vi "PH_DataViewer.set Img Op GUI elements.vi"(0 "i ref in":refnum<vi>, 2 "Img Operator Data":T2={"Instance"="N/A", "Snapshot: Date"="N/A", "Snapshot: Time"="N/A", "Calibration"={"Status"=0, "Calibration data - Version 1"={"Date"="", "Time"="", "Cam Settings"={"Serial Number"=0.0, "Gain"=0, "Brightness"=0, "Shutter"=0, "Cam Error"=FALSE, "Mode"=0}, "Background Image"={"Image"=[], "Image Error"=FALSE}, "Linear Calibration"={"Calibration Factor"=0.0, "not mm or mrad"=FALSE}, "Energy Calibration"={"Calibration Factor"=0.0, "no mJ"=FALSE}}}, "Position Analysis"={"on"=FALSE, "exp - X"=0, "exp - Y"=0, "focal length [mm]"=0.0, "Magnification"=0.0, "Delta"=0.0, "Theta"=0.0, "Tolerance"=0.0, "Type"=FALSE}, "Beam Analysis"={"on"=FALSE, "Data"={"CoG-x"=0.0, "CoG-y"=0.0, "Maj Dim"=0.0, "Min Dim"=0.0, "Ellipticity"=0.0, "Azimuth Angle [rad]"=0.0, "Azi Angle rel to Maj?"=FALSE}, "Method"=FALSE, "Steps"=3, "Factor"=3, "ROI"={"Left"=0, "Top"=0, "Right"=0, "Bottom"=0}}, "Cam Settings"={"Serial Number"=0.0, "Gain"=0, "Brightness"=0, "Shutter"=0, "Cam Info Failure"=FALSE, "Mode"=0}, "Energy"={"on"=FALSE, "expected value [mJ]"=0.0, "Tolerance [%]"=0.0, "State"=0, "Energy [mJ]"=0.0, "Unit"=""}, "Image"=[], "Final Image"={"BI Subtraction Failure"=FALSE}, "Trace Analysis"={"on"=FALSE, "Fit on"=FALSE, "Maj FWHM"=0.0, "Min FWHM"=0.0, "Maj Fit Order"=0, "Min Fit Order"=0, "No Offset"=FALSE, "Maj 99%"=0.0, "Min 99%"=0.0, "Traces"=[]}} {"Energy"."State" items=["no info", "off/false", "on/true", "Failure", "Alarm"]; "Cam Settings"."Serial Number" format="%#_12g"; "Calibration"."Calibration data - Version 1"."Cam Settings"."Serial Number" format="%#_12g"; "Calibration"."Status" items=["no info", "off/false", "on/true", "Failure", "Alarm"]}, 5 "error in (no error)":errorcluster) -> (14 "i ref out":refnum<vi>, 19 "error out":errorcluster)   [LabVIEW 2014, in "PH_DataViewer.lvlib"]
doc: "This VI indicates the results of the Image Operator"
uses:
  PH_DataViewer.lvlib
  PH_ImageOperator.Data.ctl
  PH_DataViewer.Device State.ctl
  PH_ImageCalibrator/PH_ImageCalibrator.Calibration Data - Version 1.ctl
  PH_ImageOperator/PH_ImageOperator.Beam Analysis Data.ctl
  <vilib>/vision/Image Controls.llb/IMAQ Image.ctl
  <vilib>/vision/NI_Vision_Development_Module.lvlib
  PH_ImageOperator/PH_ImageOperator.lvlib
  PH_ImageCalibrator/PH_ImageCalibrator.lvlib
panel:
  in  "Cam Settings Template":T1 caption="Settings" {"Serial Number" format="%#_15g"}
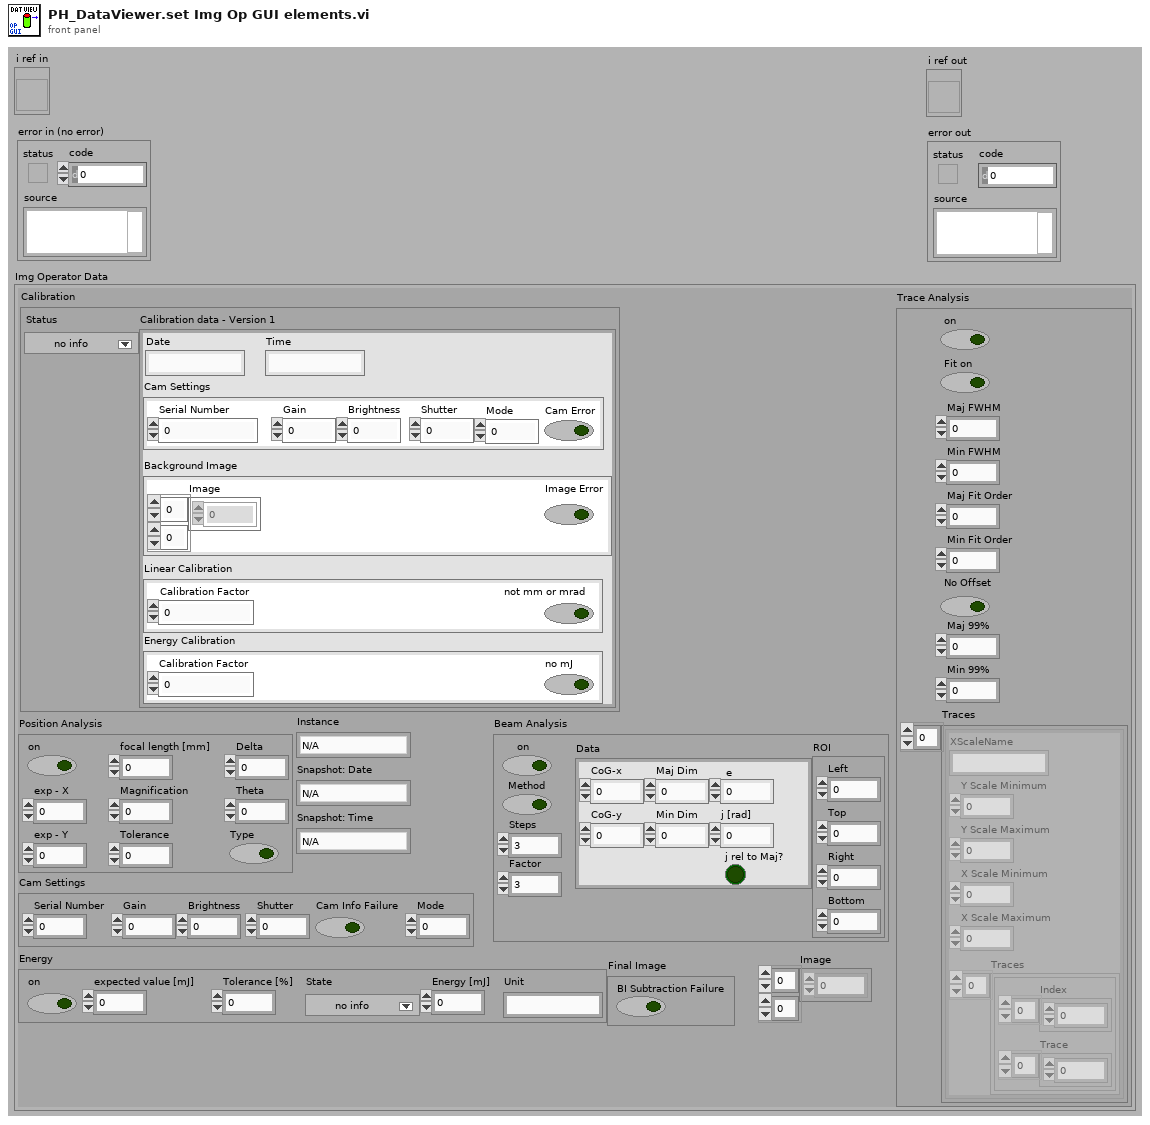
[diagram p1: front panel]
types:
  T1 = cluster{"Serial Number":dbl, "Gain":i32, "Brightness":i32, "Shutter":i32, "Mode":i32}
  T2 = typedef "PH_DataViewer.lvlib/PH_ImageOperator.Data.ctl" = cluster{"Instance":string, "Snapshot: Date":string, "Snapshot: Time":string, "Calibration":cluster{"Status":T3, "Calibration data - Version 1":T4}, "Position Analysis":cluster{"on":bool, "exp - X":i32, "exp - Y":i32, "focal length [mm]":dbl, "Magnification":dbl, "Delta":dbl, "Theta":dbl, "Tolerance":dbl, "Type":bool}, "Beam Analysis":cluster{"on":bool, "Data":T5, "Method":bool, "Steps":i32, "Factor":i32, "ROI":cluster{"Left":i32, "Top":i32, "Right":i32, "Bottom":i32}}, "Cam Settings":cluster{"Serial Number":dbl, "Gain":i32, "Brightness":i32, "Shutter":i32, "Cam Info Failure":bool, "Mode":i32}, "Energy":cluster{"on":bool, "expected value [mJ]":dbl, "Tolerance [%]":dbl, "State":T3, "Energy [mJ]":dbl, "Unit":string}, "Image":dbl[][], "Final Image":cluster{"BI Subtraction Failure":bool}, "Trace Analysis":cluster{"on":bool, "Fit on":bool, "Maj FWHM":dbl, "Min FWHM":dbl, "Maj Fit Order":i32, "Min Fit Order":i32, "No Offset":bool, "Maj 99%":dbl, "Min 99%":dbl, "Traces":cluster{"XScaleName":string, "Y Scale Minimum":sgl, "Y Scale Maximum":sgl, "X Scale Minimum":sgl, "X Scale Maximum":sgl, "Traces":cluster{"Index":sgl[], "Trace":dbl[]}[]}[]}}
  T3 = typedef "PH_DataViewer.lvlib/PH_DataViewer.Device State.ctl" = i32
  T4 = typedef "PH_ImageCalibrator.lvlib/PH_ImageCalibrator.Calibration Data - Version 1.ctl" = cluster{"Date":string, "Time":string, "Cam Settings":cluster{"Serial Number":dbl, "Gain":i32, "Brightness":i32, "Shutter":i32, "Cam Error":bool, "Mode":i32}, "Background Image":cluster{"Image":dbl[][], "Image Error":bool}, "Linear Calibration":cluster{"Calibration Factor":dbl, "not mm or mrad":bool}, "Energy Calibration":cluster{"Calibration Factor":dbl, "no mJ":bool}}
  T5 = typedef "PH_ImageOperator.lvlib/PH_ImageOperator.Beam Analysis Data.ctl" = cluster{"CoG-x":sgl, "CoG-y":sgl, "Maj Dim":dbl, "Min Dim":dbl, "Ellipticity":dbl, "Azimuth Angle [rad]":dbl, "Azi Angle rel to Maj?":bool}
  T6 = typedef "PH_DataViewer.lvlib/PH_DataViewer.i attribute.ctl" = cluster{"Images":cluster{"CAM":cluster{string, u32}, "BACKGROUND":cluster{string, u32}, "OPERATOR":cluster{string, u32}}, "Cam Operator GUI Refs":cluster{"Date Operators":refnum<vi>, "Time Operators":refnum<vi>, "Status Cali Data":refnum<vi>, "Calibration data":refnum<vi>, "Background Image":refnum<vi>, "Bg subtracted":refnum<vi>, "Op Image":refnum<vi>, "Cam Settings Operator":refnum<vi>, "Energy on":refnum<vi>, "exp Energy":refnum<vi>, "Energy":refnum<vi>, "Beam Analysis":refnum<vi>, "Analysis Type":refnum<vi>, "BA: Steps":refnum<vi>, "BA: Factor for ROI":refnum<vi>, "CoG - X":refnum<vi>, "CoG - Y":refnum<vi>, "Maj Diam":refnum<vi>, "Min Diam":refnum<vi>, "Phi":refnum<vi>, "Epsilon":refnum<vi>, "Phi rel to maj":refnum<vi>, "Position":refnum<vi>, "Position Type":refnum<vi>, "exp - X":refnum<vi>, "exp - Y":refnum<vi>, "Magni":refnum<vi>, "Foc Length":refnum<vi>, "Delta":refnum<vi>, "Theta":refnum<vi>, "Fit Gauss":refnum<vi>, "Maj Fit Order":refnum<vi>, "Min Fit Order":refnum<vi>, "Maj FWHM":refnum<vi>, "Min FWHM":refnum<vi>, "Maj 1 %":refnum<vi>, "Min 1 %":refnum<vi>}}
  T7 = cluster{"Date Operators":refnum<vi>, "Time Operators":refnum<vi>, "Status Cali Data":refnum<vi>, "Calibration data":refnum<vi>, "Background Image":refnum<vi>, "Bg subtracted":refnum<vi>, "Op Image":refnum<vi>, "Cam Settings Operator":refnum<vi>, "Energy on":refnum<vi>, "exp Energy":refnum<vi>, "Energy":refnum<vi>, "Beam Analysis":refnum<vi>, "Analysis Type":refnum<vi>, "BA: Steps":refnum<vi>, "BA: Factor for ROI":refnum<vi>, "CoG - X":refnum<vi>, "CoG - Y":refnum<vi>, "Maj Diam":refnum<vi>, "Min Diam":refnum<vi>, "Phi":refnum<vi>, "Epsilon":refnum<vi>, "Phi rel to maj":refnum<vi>, "Position":refnum<vi>, "Position Type":refnum<vi>, "exp - X":refnum<vi>, "exp - Y":refnum<vi>, "Magni":refnum<vi>, "Foc Length":refnum<vi>, "Delta":refnum<vi>, "Theta":refnum<vi>, "Fit Gauss":refnum<vi>, "Maj Fit Order":refnum<vi>, "Min Fit Order":refnum<vi>, "Maj FWHM":refnum<vi>, "Min FWHM":refnum<vi>, "Maj 1 %":refnum<vi>, "Min 1 %":refnum<vi>}
  T8 = typedef "IMAQ Image.ctl" = refnum<image>
  T9 = cluster{"Date Operators":bool, "Time Operators":bool, "Status Cali Data":bool, "Calibration data":bool, "Background Image":bool, "Bg subtracted":bool, "Op Image":bool, "Cam Settings Operator":bool, "Energy on":bool, "exp Energy":bool, "Energy":bool, "Beam Analysis":bool, "Analysis Type":bool, "BA: Steps":bool, "BA: Factor for ROI":bool, "CoG - X":bool, "CoG - Y":bool, "Maj Diam":bool, "Min Diam":bool, "Phi":bool, "Epsilon":bool, "Phi rel to maj":bool, "Position":bool, "Position Type":bool, "exp - X":bool, "exp - Y":bool, "Magni":bool, "Foc Length":bool, "Delta":bool, "Theta":bool, "Fit Gauss":bool, "Maj Fit Order":bool, "Min Fit Order":bool, "Maj FWHM":bool, "Min FWHM":bool, "Maj 1 %":bool, "Min 1 %":bool}
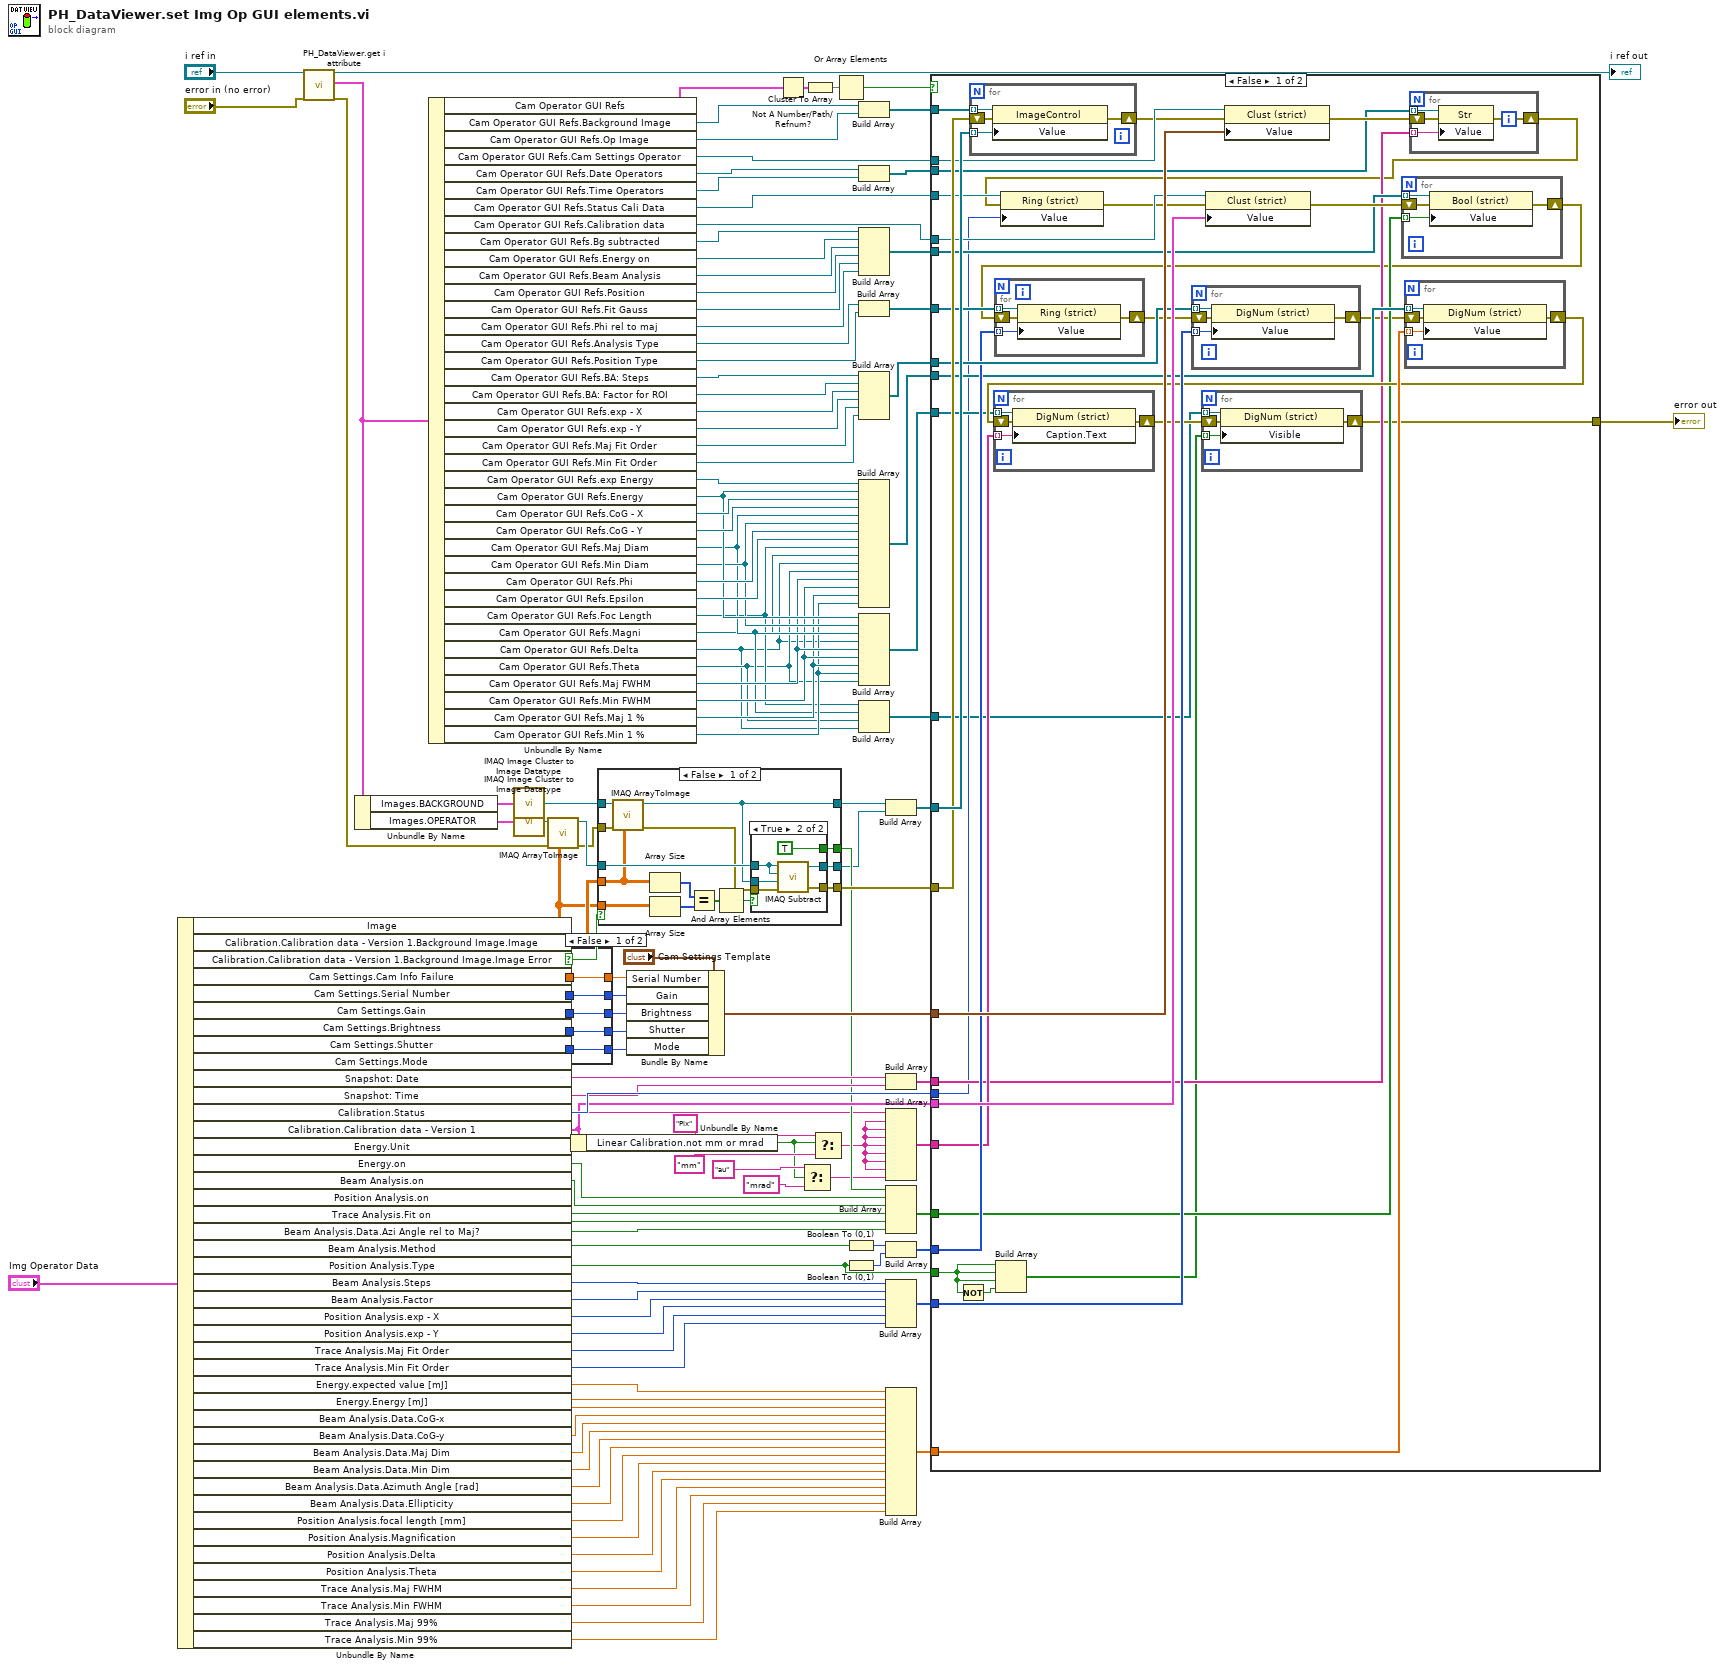
[diagram p0: block diagram]
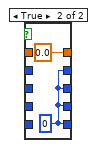
[diagram p3: hidden frame]
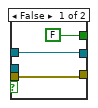
[diagram p4: hidden frame]
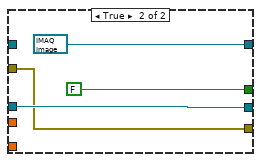
[diagram p5: hidden frame]
diagram:
  n1 = Unbundle By Name("Img Operator Data") -> ("Image"=w100:dbl[][], "Calibration.Calibration data - Version 1.Background Image.Image"=w101:dbl[][], "Calibration.Calibration data - Version 1.Background Image.Image Error"=w111:bool, "Cam Settings.Cam Info Failure"=w119:bool, "Cam Settings.Serial Number"=w120:dbl, "Cam Settings.Gain"=w122:i32, "Cam Settings.Brightness"=w124:i32, "Cam Settings.Shutter"=w126:i32, "Cam Settings.Mode"=w128:i32, "Snapshot: Date"=w64:string, "Snapshot: Time"=w65:string, "Calibration.Status"=w102:T3, "Calibration.Calibration data - Version 1"=w83:T4, "Energy.Unit"=w11:string, "Energy.on"=w77:bool, "Beam Analysis.on"=w78:bool, "Position Analysis.on"=w79:bool, "Trace Analysis.Fit on"=w80:bool, "Beam Analysis.Data.Azi Angle rel to Maj?"=w70:bool, "Beam Analysis.Method"=w96:bool, "Position Analysis.Type"=w1:bool, "Beam Analysis.Steps"=w49:i32, "Beam Analysis.Factor"=w50:i32, "Position Analysis.exp - X"=w32:i32, "Position Analysis.exp - Y"=w31:i32, "Trace Analysis.Maj Fit Order"=w30:i32, "Trace Analysis.Min Fit Order"=w29:i32, "Energy.expected value [mJ]"=w45:dbl, "Energy.Energy [mJ]"=w46:dbl, "Beam Analysis.Data.CoG-x"=w91:sgl, "Beam Analysis.Data.CoG-y"=w39:sgl, "Beam Analysis.Data.Maj Dim"=w90:dbl, "Beam Analysis.Data.Min Dim"=w89:dbl, "Beam Analysis.Data.Azimuth Angle [rad]"=w88:dbl, "Beam Analysis.Data.Ellipticity"=w87:dbl, "Position Analysis.focal length [mm]"=w24:dbl, "Position Analysis.Magnification"=w23:dbl, "Position Analysis.Delta"=w22:dbl, "Position Analysis.Theta"=w21:dbl, "Trace Analysis.Maj FWHM"=w20:dbl, "Trace Analysis.Min FWHM"=w19:dbl, "Trace Analysis.Maj 99%"=w18:dbl, "Trace Analysis.Min 99%"=w17:dbl)
  n2 = call "PH_DataViewer.get i attribute.vi"("i ref in"="i ref in", "error in (no error)"="error in (no error)") -> ("i ref out"=→"i ref out":refnum<vi>, "i attribute"=w99:T6, "error out"=w113:errorcluster)  [unwired: 15 in]
  n3 = Unbundle By Name(w99) -> ("Images.BACKGROUND"=w98:cluster{string, u32}, "Images.OPERATOR"=w97:cluster{string, u32})
  n4 = Unbundle By Name(w99) -> ("Cam Operator GUI Refs"=w110:T7, "Cam Operator GUI Refs.Background Image"=w60:refnum<vi>, "Cam Operator GUI Refs.Op Image"=w59:refnum<vi>, "Cam Operator GUI Refs.Cam Settings Operator"=w106:refnum<vi>, "Cam Operator GUI Refs.Date Operators"=w68:refnum<vi>, "Cam Operator GUI Refs.Time Operators"=w67:refnum<vi>, "Cam Operator GUI Refs.Status Cali Data"=w40:refnum<vi>, "Cam Operator GUI Refs.Calibration data"=w105:refnum<vi>, "Cam Operator GUI Refs.Bg subtracted"=w62:refnum<vi>, "Cam Operator GUI Refs.Energy on"=w75:refnum<vi>, "Cam Operator GUI Refs.Beam Analysis"=w74:refnum<vi>, "Cam Operator GUI Refs.Position"=w73:refnum<vi>, "Cam Operator GUI Refs.Fit Gauss"=w72:refnum<vi>, "Cam Operator GUI Refs.Phi rel to maj"=w69:refnum<vi>, "Cam Operator GUI Refs.Analysis Type"=w34:refnum<vi>, "Cam Operator GUI Refs.Position Type"=w35:refnum<vi>, "Cam Operator GUI Refs.BA: Steps"=w53:refnum<vi>, "Cam Operator GUI Refs.BA: Factor for ROI"=w52:refnum<vi>, "Cam Operator GUI Refs.exp - X"=w28:refnum<vi>, "Cam Operator GUI Refs.exp - Y"=w27:refnum<vi>, "Cam Operator GUI Refs.Maj Fit Order"=w26:refnum<vi>, "Cam Operator GUI Refs.Min Fit Order"=w25:refnum<vi>, "Cam Operator GUI Refs.exp Energy"=w47:refnum<vi>, "Cam Operator GUI Refs.Energy"=w43:refnum<vi>, "Cam Operator GUI Refs.CoG - X"=w94:refnum<vi>, "Cam Operator GUI Refs.CoG - Y"=w54:refnum<vi>, "Cam Operator GUI Refs.Maj Diam"=w41:refnum<vi>, "Cam Operator GUI Refs.Min Diam"=w42:refnum<vi>, "Cam Operator GUI Refs.Phi"=w93:refnum<vi>, "Cam Operator GUI Refs.Epsilon"=w92:refnum<vi>, "Cam Operator GUI Refs.Foc Length"=w6:refnum<vi>, "Cam Operator GUI Refs.Magni"=w5:refnum<vi>, "Cam Operator GUI Refs.Delta"=w3:refnum<vi>, "Cam Operator GUI Refs.Theta"=w4:refnum<vi>, "Cam Operator GUI Refs.Maj FWHM"=w16:refnum<vi>, "Cam Operator GUI Refs.Min FWHM"=w15:refnum<vi>, "Cam Operator GUI Refs.Maj 1 %"=w14:refnum<vi>, "Cam Operator GUI Refs.Min 1 %"=w13:refnum<vi>)
  n5 = call <vilib>:"IMAQ Image Cluster to Image Datatype.vi"("Image"=w98) -> ("Image (dup)"=w116:T8)
  n6 = call <vilib>:"IMAQ Image Cluster to Image Datatype.vi"("Image"=w97) -> ("Image (dup)"=w118:T8)
  n7 = call "IMAQ ArrayToImage"("Image Pixels (Float)"=w100, "error in (no error)"=w113, "Image"=w118) -> ("error out"=w114:errorcluster, "Image Out"=w117:T8)  [unwired: 7 in]
  n8 = case shown="False" w119 {
    tunnel: w120 -> [w137 _]
    tunnel: [w137 0.0 ("Serial Number")] -> w121
    tunnel: [w136 w138] -> w123
    tunnel: w122 -> [w136 _]
    tunnel: [w135 w138] -> w125
    tunnel: w124 -> [w135 _]
    tunnel: [w134 w138] -> w127
    tunnel: w126 -> [w134 _]
    tunnel: [w133 w138] -> w129
    tunnel: w128 -> [w133 _]
    frame False {
    }
    frame True {
      w138 = 0 ("Gain")
    }
  }
  n9 = Unbundle By Name(w83) -> ("Linear Calibration.not mm or mrad"=w8:bool)
  n10 = case shown="False" w111 {
    tunnel: w101 -> [w145 _]
    tunnel: [w151 T8 refnum ("Image Out")] -> w55
    tunnel: w116 -> [w153 _]
    tunnel: w117 -> [w152 w165]
    tunnel: [w150 w165] -> w57
    tunnel: [w149 FALSE] -> w61
    tunnel: w114 -> [w148 w163]
    tunnel: [w146 w163] -> w104
    tunnel: w100 -> [w144 _]
    frame False {
      n11 = call "IMAQ ArrayToImage"("Image Pixels (Float)"=w145, "error in (no error)"=w148, "Image"=w153) -> ("error out"=w147:errorcluster, "Image Out"=w151:T8)  [unwired: 7 in]
      n12 = Array Size(array=w145) -> (size(s)=w142:i32[])
      n13 = Array Size(array=w144) -> (size(s)=w143:i32[])
      n14 = Equal?(x=w142, y=w143) -> (x = y?=w141:bool[])
      n15 = And Array Elements(Boolean array=w141) -> (logical AND=w140:bool)
      n16 = case shown="True" w140 {
        tunnel: w152 -> [w155 w162]
        tunnel: w151 -> [_ w161]
        tunnel: [w155 w160] -> w150
        tunnel: [FALSE TRUE] -> w149
        tunnel: w147 -> [w154 w158]
        tunnel: [w154 w157] -> w146
        frame False {
        }
        frame True {
          n17 = call "IMAQ Subtract"("Image Src A"=w162, "Image Dst"=w162, "Image Src B"=w161, "error in (no error)"=w158) -> ("Image Dst Out"=w160:T8, "error out"=w157:errorcluster)  [unwired: 3 in]
        }
      }
    }
    frame True {
    }
  }
  n18 = Bundle By Name(cluster="Cam Settings Template", "Serial Number"=w121, "Gain"=w123, "Brightness"=w125, "Shutter"=w127, "Mode"=w129) -> (w103:T1)
  n19 = Not A Number/Path/Refnum?(number/path/refnum=w110) -> (NaN/Path/Refnum?=w108:T9)
  n20 = Select(t="au", s=w8, f="mrad") -> (s? t:f=w7:string)
  n21 = Cluster To Array(cluster=w108) -> (array=w109:bool[])
  n22 = Select(t="Pix", s=w8, f="mm") -> (s? t:f=w12:string)
  n23 = Or Array Elements(Boolean array=w109) -> (logical OR=w107:bool)
  n24 = Boolean To (0,1)(Boolean=w96) -> (0, 1=w37:i16)
  n25 = Boolean To (0,1)(Boolean=w1) -> (0, 1=w38:i16)
  n26 = Build Array(w60, w59) -> (w58:refnum<vi>[])
  n27 = Build Array(w68, w67) -> (w66:refnum<vi>[])
  n28 = Build Array(w62, w75, w74, w73, w72, w69) -> (w71:refnum<vi>[])
  n29 = Build Array(w34, w35) -> (w33:refnum<vi>[])
  n30 = Build Array(w53, w52, w28, w27, w26, w25) -> (w51:refnum<vi>[])
  n31 = Build Array(w47, w43, w94, w54, w41, w42, w93, w92, w6, w5, w3, w4, w16, w15, w14, w13) -> (w85:refnum<vi>[])
  n32 = Build Array(w43, w42, w41, w3, w16, w15, w14, w13, w4) -> (w84:refnum<vi>[])
  n33 = Build Array(w6, w5, w4, w3) -> (w2:refnum<vi>[])
  n34 = Build Array(w55, w57) -> (w56:T8[])
  n35 = Build Array(w64, w65) -> (w63:string[])
  n36 = Build Array(w11, w12, w12, w12, w12, w12, w12, w12, w7) -> (w44:string[])
  n37 = Build Array(w61, w77, w78, w79, w80, w70) -> (w76:bool[])
  n38 = Build Array(w37, w38) -> (w36:i16[])
  n39 = Build Array(w49, w50, w32, w31, w30, w29) -> (w48:i32[])
  n40 = Build Array(w45, w46, w91, w39, w90, w89, w88, w87, w24, w23, w22, w21, w20, w19, w18, w17) -> (w86:dbl[])
  n41 = case shown="False" w107 {
    tunnel: w58 -> [w177 _]
    tunnel: w106 -> [w200 _]
    tunnel: w40 -> [w197 _]
    tunnel: w105 -> [w196 _]
    tunnel: w56 -> [w202 _]
    tunnel: w104 -> [w201 w235]
    tunnel: w103 -> [w199 _]
    tunnel: w102 -> [w174 _]
    tunnel: w83 -> [w195 _]
    tunnel: w48 -> [w189 _]
    tunnel: w33 -> [w193 _]
    tunnel: w51 -> [w192 _]
    tunnel: w36 -> [w190 _]
    tunnel: [w171 w235] -> w95
    tunnel: w86 -> [w188 _]
    tunnel: w85 -> [w187 _]
    tunnel: w84 -> [w185 _]
    tunnel: w44 -> [w184 _]
    tunnel: w76 -> [w182 _]
    tunnel: w71 -> [w183 _]
    tunnel: w66 -> [w181 _]
    tunnel: w63 -> [w180 _]
    tunnel: w2 -> [w170 _]
    tunnel: w1 -> [w169 _]
    frame False {
      n42 = Not(x=w169) -> (.not. x?=w168:bool)
      n43 = for {
        tunnel: w202 -> [w218] mode=indexing
        shift-right: [w216] -> w179
        shift-left: w201 -> [w217]
        tunnel: w177 -> [w215] mode=indexing
        n44 = property class="ImageControl"(reference=w215, error in=w217, "Value"=w218) -> (error out=w216:errorcluster)  [unwired: 1 out]
      }
      n45 = Build Array(w169, w169, w169, w168) -> (w167:bool[])
      n46 = property class="Clust (strict)"(reference=w200, error in=w179, "Value"=w199) -> (error out=w198:errorcluster)  [unwired: 1 out]
      n47 = for {
        tunnel: w180 -> [w221] mode=indexing
        shift-right: [w220] -> w173
        shift-left: w198 -> [w222]
        tunnel: w181 -> [w219] mode=indexing
        n48 = property class="Str"(reference=w219, error in=w222, "Value"=w221) -> (error out=w220:errorcluster)  [unwired: 1 out]
      }
      n49 = property class="Ring (strict)"(reference=w197, error in=w173, "Value"=w174) -> (error out=w178:errorcluster)  [unwired: 1 out]
      n50 = property class="Clust (strict)"(reference=w196, error in=w178, "Value"=w195) -> (error out=w194:errorcluster)  [unwired: 1 out]
      n51 = for {
        shift-right: [w226] -> w175
        shift-left: w194 -> [w225]
        tunnel: w183 -> [w224] mode=indexing
        tunnel: w182 -> [w223] mode=indexing
        n52 = property class="Bool (strict)"(reference=w224, error in=w225, "Value"=w223) -> (error out=w226:errorcluster)  [unwired: 1 out]
      }
      n53 = for {
        tunnel: w193 -> [w210] mode=indexing
        tunnel: w190 -> [w208] mode=indexing
        shift-right: [w209] -> w191
        shift-left: w175 -> [w207]
        n54 = property class="Ring (strict)"(reference=w210, error in=w207, "Value"=w208) -> (error out=w209:errorcluster)  [unwired: 1 out]
      }
      n55 = for {
        tunnel: w192 -> [w214] mode=indexing
        tunnel: w189 -> [w212] mode=indexing
        shift-right: [w211] -> w176
        shift-left: w191 -> [w213]
        n56 = property class="DigNum (strict)"(reference=w214, error in=w213, "Value"=w212) -> (error out=w211:errorcluster)  [unwired: 1 out]
      }
      n57 = for {
        shift-right: [w233] -> w186
        shift-left: w176 -> [w234]
        tunnel: w187 -> [w232] mode=indexing
        tunnel: w188 -> [w231] mode=indexing
        n58 = property class="DigNum (strict)"(reference=w232, error in=w234, "Value"=w231) -> (error out=w233:errorcluster)  [unwired: 1 out]
      }
      n59 = for {
        shift-right: [w229] -> w172
        shift-left: w186 -> [w230]
        tunnel: w185 -> [w228] mode=indexing
        tunnel: w184 -> [w227] mode=indexing
        n60 = property class="DigNum (strict)"(reference=w228, error in=w230, "Caption.Text"=w227) -> (error out=w229:errorcluster)  [unwired: 1 out]
      }
      n61 = for {
        shift-right: [w205] -> w171
        shift-left: w172 -> [w206]
        tunnel: [w203] -> _ mode=indexing
        tunnel: w167 -> [w204] mode=indexing
        tunnel: w170 -> [w203] mode=indexing
        n62 = property class="DigNum (strict)"(reference=w203, error in=w206, "Visible"=w204) -> (error out=w205:errorcluster)  [unwired: 1 out]
      }
    }
    frame True {
    }
  }
  "error out" <- w95
